vi "set_socket_timeout.vi"(0 "zmq_mlt in":refnum<class "zmq_multipart_lib.lvclass">, 5 "recv_timeout_ms":dbl, 7 "send_timeout_ms":dbl, 11 "error in (no error)":errorcluster) -> (4 "zmq_mlt out":refnum<class "zmq_multipart_lib.lvclass">, 15 "error out":errorcluster)   [LabVIEW 2019, in "zmq_multipart_lib.lvlib" / "zmq_multipart_lib.lvclass"]
uses:
  zmq_multipart_lib.lvclass
  <vilib>/addons/zeromq/zmq_socket.lvclass
  <vilib>/addons/zeromq/socket_options.ctl
  <vilib>/addons/zeromq/zeromq.lvlib
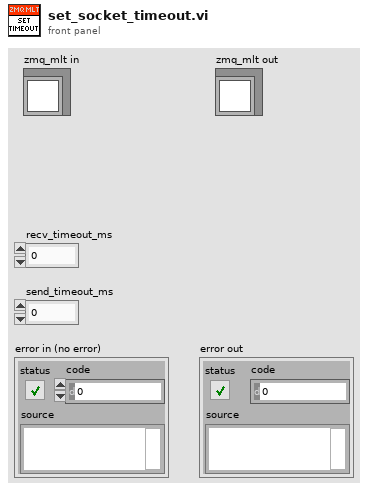
[diagram p1: front panel]
types:
  T1 = typedef "zeromq.lvlib/socket_options.ctl" = enum8{"NONE", "ZMQ_HWM", "<2>", "ZMQ_SWAP", "ZMQ_AFFINITY", "ZMQ_IDENTITY", "ZMQ_SUBSCRIBE", "ZMQ_UNSUBSCRIBE", "ZMQ_RATE", "ZMQ_RECOVERY_IVL", "ZMQ_MCAST_LOOP", "ZMQ_SNDBUF", "ZMQ_RCVBUF", "ZMQ_RCVMORE", "ZMQ_FD", "ZMQ_EVENTS", "ZMQ_TYPE", "ZMQ_LINGER", "ZMQ_RECONNECT_IVL", "ZMQ_BACKLOG", "ZMQ_RECOVERY_IVL_MSEC", "ZMQ_RECONNECT_IVL_MAX", "ZMQ_MAXMSGSIZE", "ZMQ_SNDHWM", "ZMQ_RCVHWM", "ZMQ_MULTICAST_HOPS", "<26>", "ZMQ_RCVTIMEO", "ZMQ_SNDTIMEO", "<29>", "<30>", "ZMQ_IPV4ONLY", "ZMQ_LAST_ENDPOINT", "ZMQ_ROUTER_MANDATORY", "ZMQ_TCP_KEEPALIVE", "ZMQ_TCP_KEEPALIVE_CNT", "ZMQ_TCP_KEEPALIVE_IDLE", "ZMQ_TCP_KEEPALIVE_INTVL", "ZMQ_TCP_ACCEPT_FILTER", "ZMQ_DELAY_ATTACH_ON_CONNECT", "ZMQ_XPUB_VERBOSE"}
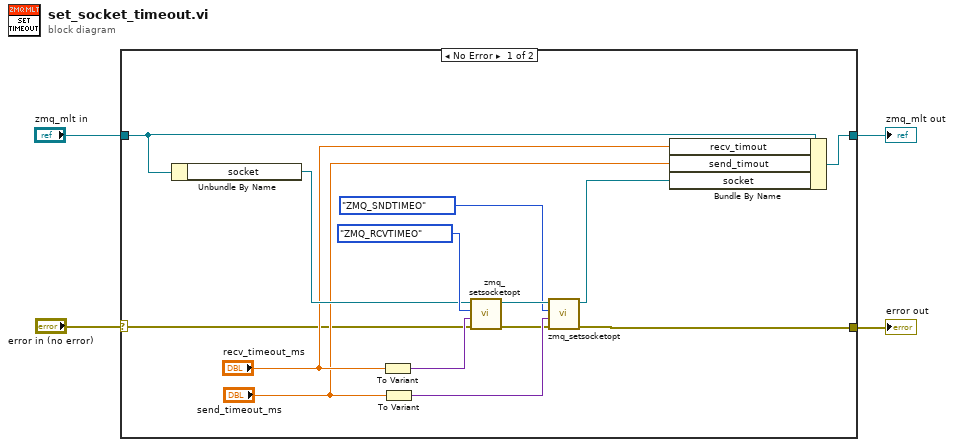
[diagram p0: block diagram]
diagram:
  n1 = case shown="No Error" "error in (no error)" {
    selector: "error in (no error)" -> [w5 w20]
    tunnel: [w13 w20] -> w4
    tunnel: "zmq_mlt in" -> [w11 w19]
    tunnel: [w9 w19] -> w2
    frame No Error {
      n2 = Unbundle By Name(w11) -> ("socket"=w10:refnum<class "zmq_socket.lvclass">)
      n3 = To Variant(anything="recv_timeout_ms") -> (Variant=w17:variant)
      n4 = To Variant(anything="send_timeout_ms") -> (Variant=w18:variant)
      n5 = call <vilib>:"zmq_setsocketopt.vi"("error in"=w5, "value"=w17, "option"=socket_options."ZMQ_RCVTIMEO", "socket in"=w10) -> ("error out"=w12:errorcluster, "socket out"=w16:refnum<class "zmq_socket.lvclass">)  [unwired: 2 in]
      n6 = call <vilib>:"zmq_setsocketopt.vi"("error in"=w12, "value"=w18, "option"=socket_options."ZMQ_SNDTIMEO", "socket in"=w16) -> ("error out"=w13:errorcluster, "socket out"=w8:refnum<class "zmq_socket.lvclass">)  [unwired: 2 in]
      n7 = Bundle By Name(cluster=w11, "recv_timout"="recv_timeout_ms", "send_timout"="send_timeout_ms", "socket"=w8) -> (w9:refnum<class "zmq_multipart_lib.lvclass">)
    }
    frame Error {
    }
  }
  "error out" <- w4
  "zmq_mlt out" <- w2
